vi "@destroy.vi"(8 "error in (no error)":errorcluster, 11 "dotnet_system_exec in":refnum<class "dotnet_system_exec.lvclass">) -> (0 "error out":errorcluster, 3 "dotnet_system_exec out":refnum<class "dotnet_system_exec.lvclass">)   [LabVIEW 2015, in "dotnet_system_exec.lvclass"]
doc: "Stops the .NET System Process and destroy the necessary references."
uses:
  dotnet_system_exec.lvclass
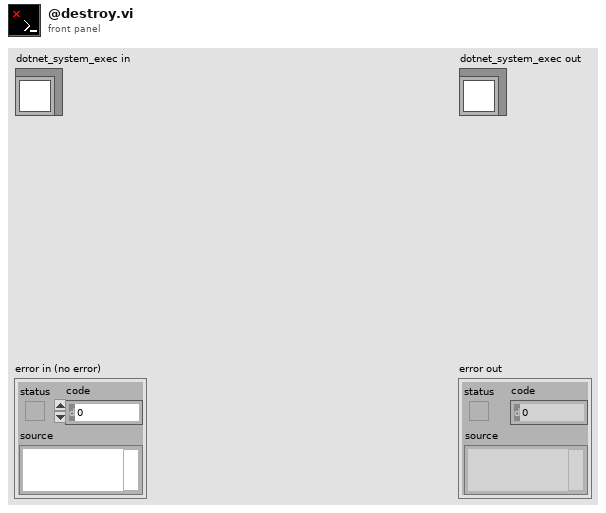
[diagram p1: front panel]
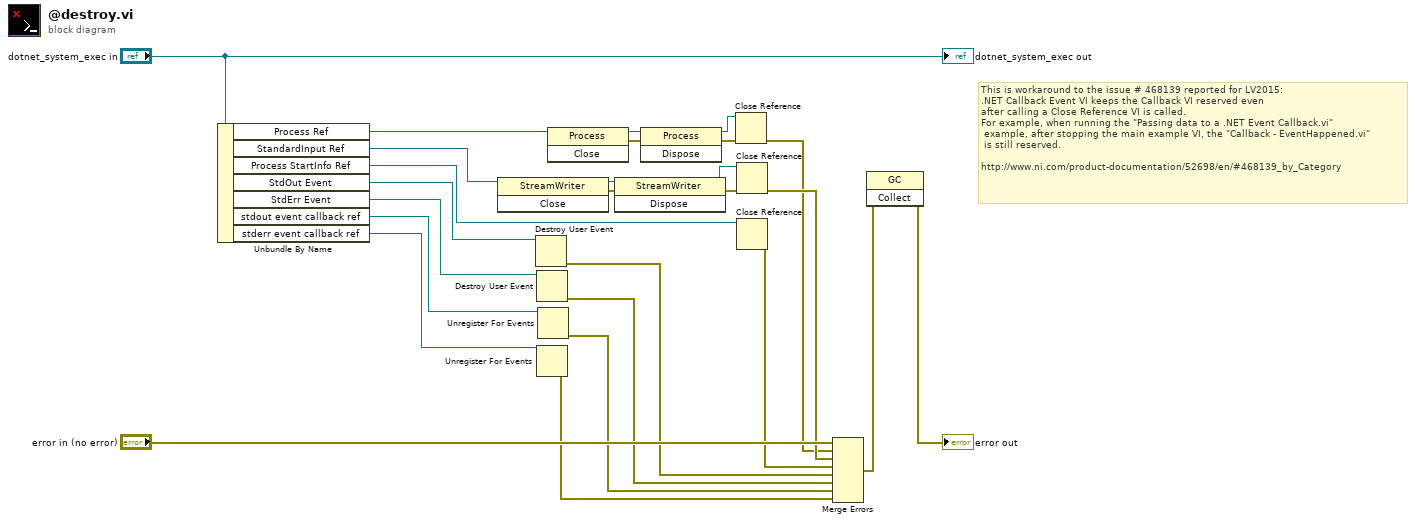
[diagram p0: block diagram]
diagram:
  # "This is workaround to the issue # 468139 reported for LV2015:\n.NET Callback Event VI keeps the Callback VI reserved even \nafter calling a Close Reference VI is called.\nFor example, when running the \"Passing data to a .NET Event Callback.vi\"\n example, after stopping the main example VI, the \"Callback - EventHappened.vi\"\n is still reserved.\n\nhttp://www.ni.com/product-documentation/52698/en/#468139_by_Category"
  n1 = Unbundle By Name("dotnet_system_exec in") -> ("Process Ref"=w4:refnum<k24>, "StandardInput Ref"=w15:refnum<k24>, "Process StartInfo Ref"=w14:refnum<k24>, "StdOut Event"=w12:refnum<user-event>, "StdErr Event"=w11:refnum<user-event>, "stdout event callback ref"=w8:refnum<k27>, "stderr event callback ref"=w7:refnum<k27>)
  n2 = invoke class="StreamWriter" method="Close"(reference=w15) -> (reference out=w24:refnum<k24>, error out=w23:errorcluster)  [unwired: 2 in, 1 out]
  n3 = Destroy User Event(user event=w12) -> (error out=w10:errorcluster)  [unwired: 1 in]
  n4 = Destroy User Event(user event=w11) -> (error out=w9:errorcluster)  [unwired: 1 in]
  n5 = Unregister For Events(event registration refnum=w7) -> (error out=w5:errorcluster)  [unwired: 1 in]
  n6 = Unregister For Events(event registration refnum=w8) -> (error out=w6:errorcluster)  [unwired: 1 in]
  n7 = invoke class="Process" method="Close"(reference=w4) -> (reference out=w20:refnum<k24>, error out=w19:errorcluster)  [unwired: 2 in, 1 out]
  n8 = invoke class="StreamWriter" method="Dispose"(reference=w24, error in=w23) -> (reference out=w21:refnum<k24>, error out=w22:errorcluster)  [unwired: 1 in, 1 out]
  n9 = invoke class="Process" method="Dispose"(reference=w20, error in=w19) -> (reference out=w17:refnum<k24>, error out=w18:errorcluster)  [unwired: 1 in, 1 out]
  n10 = Close Reference(reference=w17, error in (no error)=w18) -> (error out=w3:errorcluster)
  n11 = Close Reference(reference=w21, error in (no error)=w22) -> (error out=w16:errorcluster)
  n12 = Close Reference(reference=w14) -> (error out=w13:errorcluster)  [unwired: 1 in]
  n13 = Merge Errors("error in (no error)", w3, w16, w13, w10, w9, w6, w5) -> (w2:errorcluster)
  n14 = invoke class="GC" method="Collect"(error in=w2) -> (error out=→"error out":errorcluster)  [unwired: 2 in, 2 out]
  "dotnet_system_exec out" <- "dotnet_system_exec in"
